vi "Write Duty Cycle.vi"(0 "Triangle in":refnum<class "SV Triangle.lvclass">, 5 "duty cycle [%]":dbl, 11 "error in (no error)":errorcluster) -> (4 "Triangle out":refnum<class "SV Triangle.lvclass">, 15 "error out":errorcluster)   [LabVIEW 2017, in "SV Triangle.lvclass"]
uses:
  <vilib>/addons/_NISVFA/_Generation/Signal Generation/SV Triangle/SV Triangle.lvclass
  <vilib>/addons/_NISVFA/_Generation/Signal Generation/SV Triangle/SV Triangle.lvclass/SV Triangle.ctl
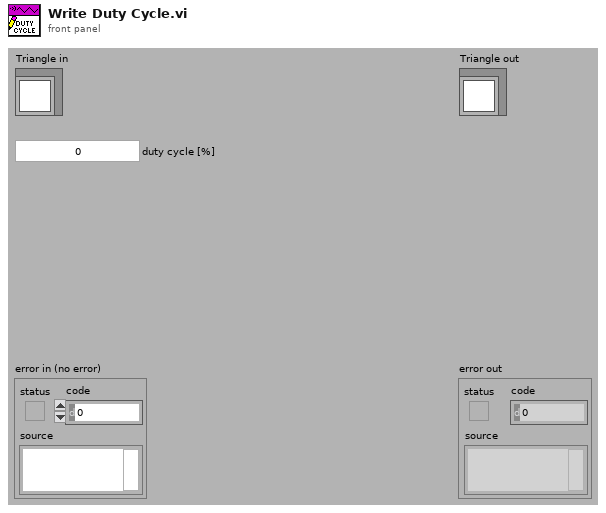
[diagram p1: front panel]
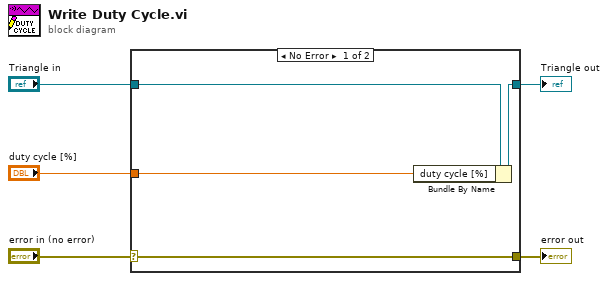
[diagram p0: block diagram]
diagram:
  n1 = case shown="No Error" "error in (no error)" {
    selector: "error in (no error)" -> [w9 w10]
    tunnel: [w9 w10] -> w4
    tunnel: [w7 w11] -> w2
    tunnel: "Triangle in" -> [w8 w11]
    tunnel: "duty cycle [%]" -> [w6 _]
    frame No Error {
      n2 = Bundle By Name(cluster=w8, "duty cycle [%]"=w6) -> (w7:refnum<class "SV Triangle.lvclass">)
    }
    frame Error {
    }
  }
  "error out" <- w4
  "Triangle out" <- w2
